vi "target_distance_angle.vi"() -> ()   [LabVIEW 2025]
uses:
  <vilib>/Rock Robotics/WPI/ThirdParty/JAS_Junk/TrajLib/TypeDef/TRANSLATION2D.ctl
  <vilib>/Rock Robotics/WPI/ThirdParty/JAS_Junk/TrajLib/TypeDef/ROTATION2D.ctl
  <vilib>/Rock Robotics/WPI/ThirdParty/JAS_Junk/TrajLib/MathUtil_InputModulus.vi
  <vilib>/Rock Robotics/WPI/ThirdParty/JAS_Junk/TrajLib/Translation2d_GetXY.vi
  <vilib>/Rock Robotics/WPI/ThirdParty/JAS_Junk/TrajLib/Rotation2d_CreateXY.vi
  <vilib>/Rock Robotics/WPI/ThirdParty/JAS_Junk/TrajLib/Rotation2d_UnaryMinus.vi
  <vilib>/Rock Robotics/WPI/ThirdParty/JAS_Junk/TrajLib/Rotation2d_RotateBy.vi
  <vilib>/Rock Robotics/WPI/ThirdParty/JAS_Junk/TrajLib/Util_CalcDist.vi
  SubVIs/TargetCalcGlobals.vi
  <vilib>/Rock Robotics/WPI/ThirdParty/JAS_Junk/TrajLib/Trajectory_Library.lvlib
panel:
  out "desired turret angle":T1 {"SIN" format="%13.4f"; "COS" format="%13.4f"; "VALUE" format="%13.4f"}
  out "Robot to Target angle":T1={"VALUE"=0.0, "COS"=1.0, "SIN"=0.0} {"SIN" format="%13.4f"; "COS" format="%13.4f"; "VALUE" format="%13.4f"}
  out "Dist M":dbl
  out "Robot Pos":T2 {"Y" format="%14.3f"; "X" format="%14.3f"}
  out "Turret Pos":T2 {"Y" format="%14.3f"; "X" format="%14.3f"}
  out "Angle To Ball (Degrees)":dbl
  out "Distance To Ball (Inches)":dbl
  in  "Y  INCHES - BALL":dbl=150.0
  in  "X INCHES - BALL":dbl=200.0
  in  "ORIENTATION - DEG":dbl=42.0
  in  "Y  INCHES":dbl=150.0
  in  "X INCHES":dbl=46.0
  # "ROBOT"
  # "BALL"
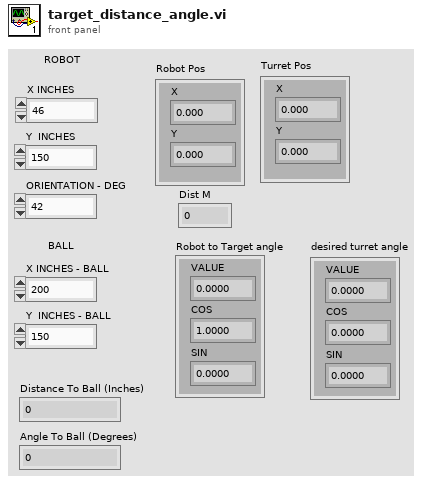
[diagram p1: front panel]
types:
  T1 = typedef "Trajectory_Library.lvlib/ROTATION2D.ctl" = cluster{"VALUE":dbl, "COS":dbl, "SIN":dbl}
  T2 = typedef "Trajectory_Library.lvlib/TRANSLATION2D.ctl" = cluster{"X":dbl, "Y":dbl}
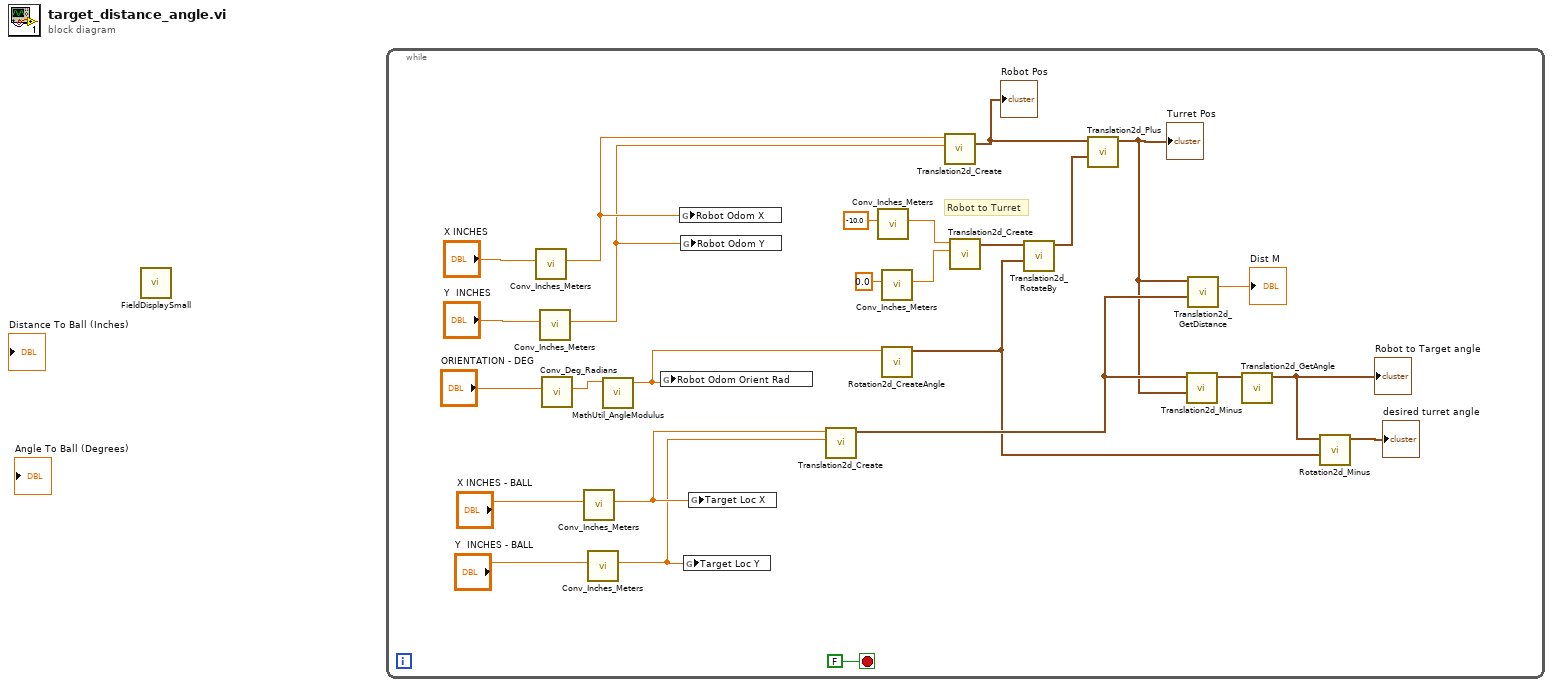
[diagram p0: block diagram]
diagram:
  n1 = call "FieldDisplaySmall.vi"() -> ()  [unwired: 1 in]
  n2 = while {
    stop <- FALSE stop-if-true
    # "Robot to Turret"
    n3 = call <vilib>:"Conv_Inches_Meters.vi"("INCH"="X INCHES") -> ("Meters"=w13:dbl)  [unwired: 10 in]
    n4 = call <vilib>:"Conv_Inches_Meters.vi"("INCH"="Y  INCHES") -> ("Meters"=w12:dbl)  [unwired: 10 in]
    n5 = call <vilib>:"Conv_Deg_Radians.vi"("Degress"="ORIENTATION - DEG") -> ("Radians"=w25:dbl)  [unwired: 10 in]
    n6 = call <vilib>:"Conv_Inches_Meters.vi"("INCH"="X INCHES - BALL") -> ("Meters"=w9:dbl)  [unwired: 10 in]
    n7 = call <vilib>:"Conv_Inches_Meters.vi"("INCH"="Y  INCHES - BALL") -> ("Meters"=w8:dbl)  [unwired: 10 in]
    n8 = call <vilib>:"MathUtil_AngleModulus.vi"("InputAngle"=w25) -> ("ModulsAngle"=w16:dbl)  [unwired: 10 in]
    n9 = global write "TargetCalcGlobals.vi" "Robot Odom Orient Rad"(w16) -> ()
    n10 = global write "TargetCalcGlobals.vi" "Robot Odom X"(w13) -> ()
    n11 = global write "TargetCalcGlobals.vi" "Robot Odom Y"(w12) -> ()
    n12 = global write "TargetCalcGlobals.vi" "Target Loc Y"(w8) -> ()
    n13 = global write "TargetCalcGlobals.vi" "Target Loc X"(w9) -> ()
    n14 = call <vilib>:"Translation2d_Create.vi"("Y"=w8, "X"=w9) -> ("TRANSLATION"=w5:T2)  [unwired: 9 in]
    n15 = call <vilib>:"Conv_Inches_Meters.vi"("INCH"=-10.0) -> ("Meters"=w21:dbl)  [unwired: 10 in]
    n16 = call <vilib>:"Conv_Inches_Meters.vi"("INCH"=0.0) -> ("Meters"=w20:dbl)  [unwired: 10 in]
    n17 = call <vilib>:"Rotation2d_CreateAngle.vi"("Angle"=w16) -> ("ROTATION"=w2:T1)  [unwired: 10 in]
    n18 = call <vilib>:"Translation2d_Create.vi"("Y"=w12, "X"=w13) -> ("TRANSLATION"=w15:T2)  [unwired: 9 in]
    "Robot Pos" <- w15
    n19 = call <vilib>:"Translation2d_Create.vi"("Y"=w20, "X"=w21) -> ("TRANSLATION"=w17:T2)  [unwired: 9 in]
    n20 = call <vilib>:"Translation2d_RotateBy.vi"("other Rotation"=w2, "In Translation"=w17) -> ("Out Translation"=w14:T2)  [unwired: 9 in]
    n21 = call <vilib>:"Translation2d_Plus.vi"("other Translation"=w14, "In Translation"=w15) -> ("Out Translation"=w4:T2)  [unwired: 9 in]
    "Turret Pos" <- w4
    n22 = call <vilib>:"Translation2d_Minus.vi"("other Translation"=w4, "In Translation"=w5) -> ("Out Translation"=w6:T2)  [unwired: 9 in]
    n23 = call <vilib>:"Translation2d_GetDistance.vi"("other Translation"=w5, "In Translation"=w4) -> ("Distance"=→"Dist M":dbl)  [unwired: 9 in]
    n24 = call <vilib>:"Translation2d_GetAngle.vi"("In Translation"=w6) -> ("Angle_Rotation2d"=w3:T1)  [unwired: 10 in]
    "Robot to Target angle" <- w3
    n25 = call <vilib>:"Rotation2d_Minus.vi"("other ROTATION"=w2, "in ROTATION"=w3) -> ("out ROTATION"=→"desired turret angle":T1)  [unwired: 9 in]
  }
